vi "Data Acq Text In.vi"(1 "command text in":string[](array[string])=["N/A", "Magent PS", "N/A", "Set Field", "Set Field to 2.0000E+0 @ 0.0000T /min, no wait , extra 0 sec wait", "N/A", "N/A", "", "1", "0", "N/A", "2.000000", "0.000000", "N/A", "N/A", "N/A", "N/A", "N/A", "N/A", "N/A", "N/A", "N/A", "N/A", "N/A", "N/A", "N/A", "N/A", "N/A", "N/A", "N/A", "N/A", "N/A", "N/A", "N/A"]) -> (0 "Data Acq":T1={"New/Stop File"=enum."New File", "Comments Option"=FALSE, "Comments"="", "extra wait"=5} {"extra wait" min=0})   [LabVIEW 2020]
uses:
  Data Acq.ctl
panel:
  # "AND wait extra"
  # "seconds"
  # "Advanced Control"
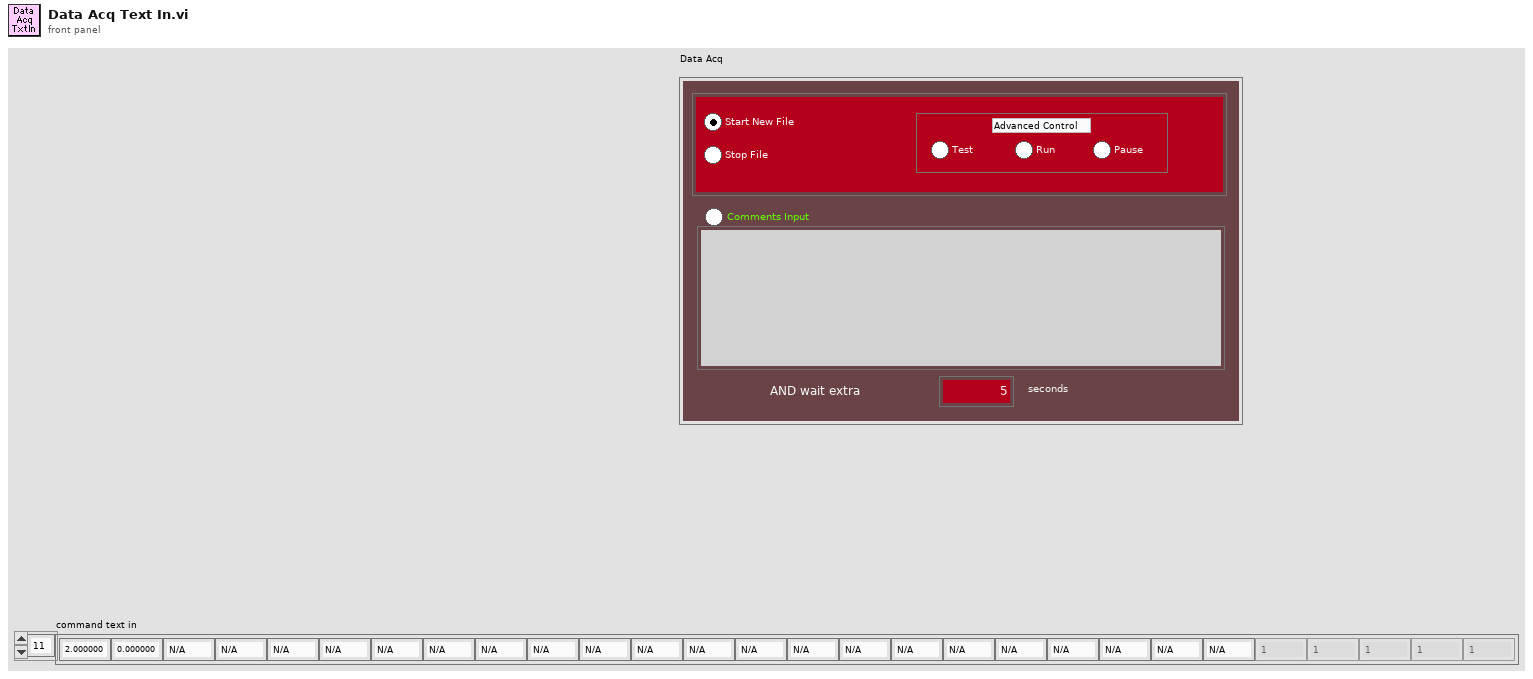
[diagram p1: front panel]
types:
  T1 = typedef "Data Acq.ctl" = cluster{"New/Stop File":enum32{"New File", "Stop FIle", "Test", "Run", "Pause"}, "Comments Option":bool, "Comments":string, "extra wait":i32}
  T2 = cluster{"command text in[0]":string, "command text in[1]":string, "command text in[2]":string, "command text in[3]":string, "command text in[4]":string, "command text in[5]":string, "command text in[6]":string, "command text in[7]":string, "command text in[8]":string, "command text in[9]":string, "command text in[10]":string, "command text in[11]":string, "command text in[12]":string, "command text in[13]":string, "command text in[14]":string, "command text in[15]":string, "command text in[16]":string, "command text in[17]":string, "command text in[18]":string, "command text in[19]":string, "command text in[20]":string, "command text in[21]":string, "command text in[22]":string, "command text in[23]":string, "command text in[24]":string, "command text in[25]":string}
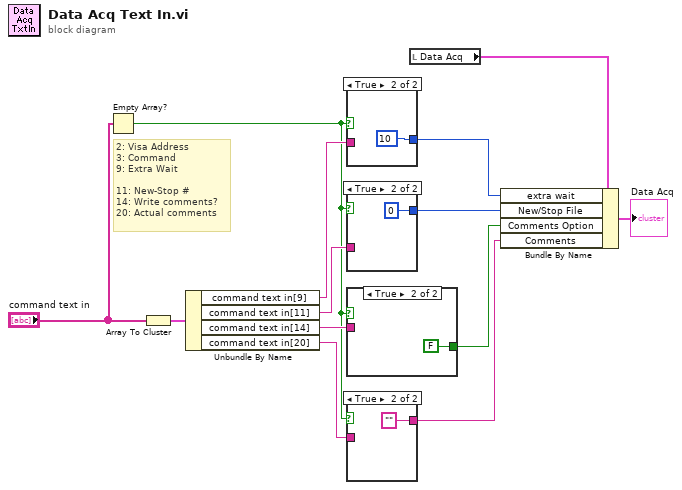
[diagram p0: block diagram]
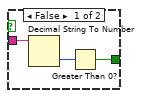
[diagram p3: hidden frame]
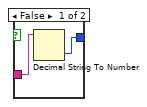
[diagram p4: hidden frame]
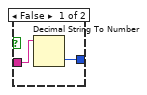
[diagram p5: hidden frame]
diagram:
  # "2: Visa Address\n3: Command\n9: Extra Wait\n\n11: New-Stop #\n14: Write comments?\n20: Actual comments"
  n1 = Empty Array?(array="command text in") -> (empty?=w6:bool)
  n2 = Array To Cluster(array="command text in") -> (cluster=w13:T2)
  n3 = Unbundle By Name(w13) -> ("command text in[9]"=w11:string, "command text in[11]"=w10:string, "command text in[14]"=w9:string, "command text in[20]"=w5:string)
  n4 = case shown="True" w6 {
    tunnel: w11 -> [w15 _]
    tunnel: [w14 u16 10 ("Value (Signaling)")] -> w4
    frame False {
      n5 = Decimal String To Number(string=w15) -> (number=w14:i32)  [unwired: 2 in, 1 out]
    }
    frame True {
    }
  }
  n6 = case shown="True" w6 {
    tunnel: w10 -> [w18 _]
    tunnel: [w17 0] -> w3
    frame False {
      n7 = Decimal String To Number(string=w18) -> (number=w17:i32)  [unwired: 2 in, 1 out]
    }
    frame True {
    }
  }
  n8 = case shown="True" w6 {
    tunnel: w9 -> [w22 _]
    tunnel: [w21 FALSE] -> w2
    frame False {
      n9 = Decimal String To Number(string=w22) -> (number=w20:i32)  [unwired: 2 in, 1 out]
      n10 = Greater Than 0?(x=w20) -> (x > 0?=w21:bool)
    }
    frame True {
    }
  }
  n11 = case shown="True" w6 {
    tunnel: [w24 ""] -> w1
    tunnel: w5 -> [w24 _]
    frame False {
    }
    frame True {
    }
  }
  n12 = local read "Data Acq"() -> (w8:T1)
  n13 = Bundle By Name(cluster=w8, "extra wait"=w4, "New/Stop File"=w3, "Comments Option"=w2, "Comments"=w1) -> (→"Data Acq":T1)
